vi "Get User Attribute Value.vi"(0 "iUser Configuration Manager DVR":refnum<data-value>, 5 "Username":string, 7 "Attribute Name":string, 11 "error in":errorcluster) -> (4 "dup iUser Configuration Manager DVR":refnum<data-value>, 6 "Attribute Value":variant, 8 "Found":bool, 15 "error out":errorcluster)   [LabVIEW 2017, in "User Configuration Manager.lvlib" / "By Ref.lvlib"]
doc: "Gets the attribute's value specified by attribute name from the user specified by user name."
uses:
  <vilib>/gpm_packages/@cs/user-manager/Source/User Configuration Manager Ref/By Ref.lvlib
  <vilib>/gpm_packages/@cs/user-manager/Source/iUser Configuration Manager/iUser Configuration Manager.lvclass
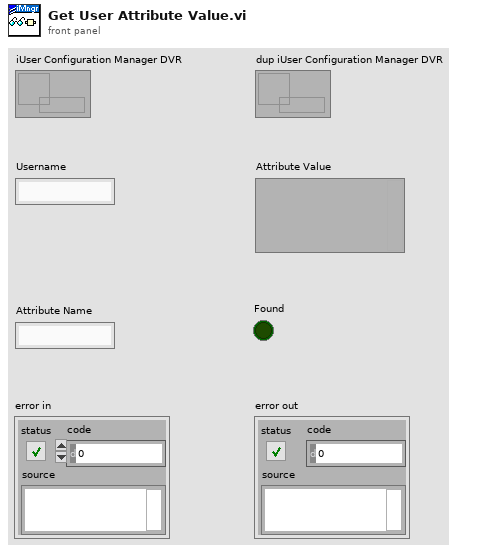
[diagram p1: front panel]
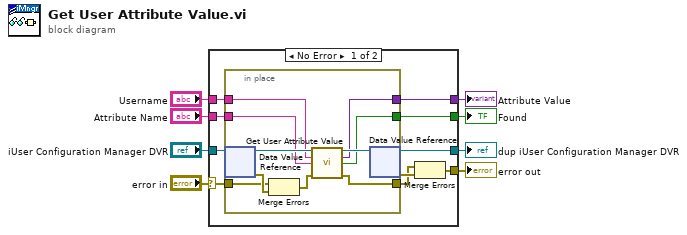
[diagram p0: block diagram]
diagram:
  n1 = case shown="No Error" "error in" {
    selector: "error in" -> [w16 w30]
    tunnel: "iUser Configuration Manager DVR" -> [w18 w29]
    tunnel: [w17 w30] -> w7
    tunnel: [w13 w29] -> w5
    tunnel: "Username" -> [w12 _]
    tunnel: "Attribute Name" -> [w11 _]
    tunnel: [w10 _] -> w2
    tunnel: [w9 _] -> w1
    frame No Error {
      n2 = in-place "IPES" {
        in-place-border: [w22] -> w14
        in-place-border: w16 -> [w27]
        in-place-border: w12 -> [w21]
        in-place-border: w11 -> [w19]
        in-place-border: [w24] -> w10
        in-place-border: [w23] -> w9
        n3 = in-place-dvr #1(w18) -> (w26:refnum<class "iUser Configuration Manager.lvclass">, w28:errorcluster)
        n4 = Merge Errors(w27, w28) -> (w20:errorcluster)
        n5 = call-dynamic "Get User Attribute Value.vi"("iUser Configuration Manager in"=w26, "Username"=w21, "Attribute Name"=w19, "error in (no error)"=w20) -> ("iUser Configuration Manager out"=w25:refnum<class "iUser Configuration Manager.lvclass">, "Attribute Value"=w24:variant, "Found"=w23:bool, "error out"=w22:errorcluster)  [unwired: 8 in]
        n6 = in-place-dvr #1(w25) -> (w13:refnum<data-value>, w15:errorcluster)
      }
      n7 = Merge Errors(w14, w15) -> (w17:errorcluster)
    }
    frame Error {
    }
  }
  "error out" <- w7
  "dup iUser Configuration Manager DVR" <- w5
  "Attribute Value" <- w2
  "Found" <- w1
